vi "GetXL_SheetNames.vi"(8 "error in (no error)":errorcluster, 11 "Refnum Cluster In":T1) -> (0 "error out":errorcluster, 2 "SheetNames(\"\")":string[](array[string]), 3 "Refnum Cluster Out":T1)   [LabVIEW 2015]
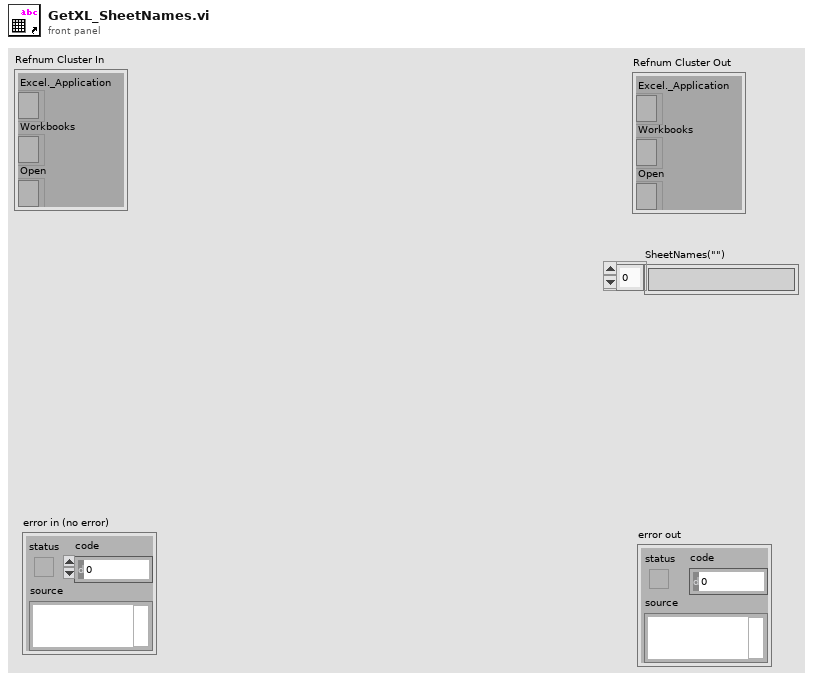
[diagram p1: front panel]
types:
  T1 = cluster{"Excel._Application":refnum<k7>, "Workbooks":refnum<k7>, "Open":refnum<k7>}
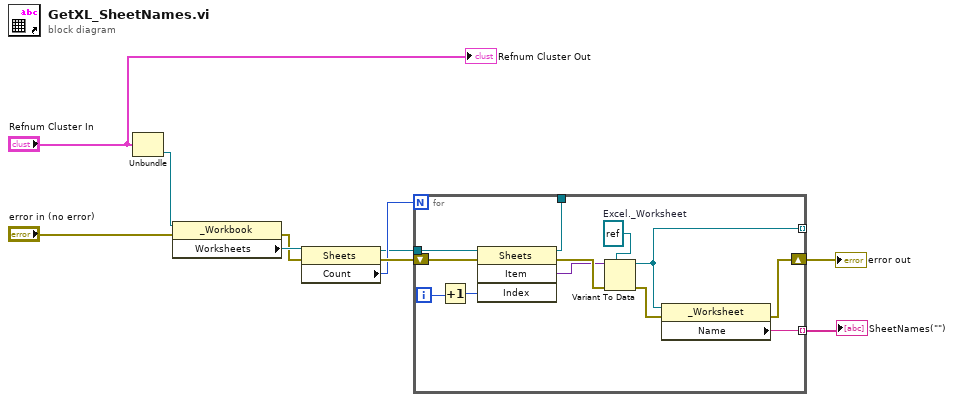
[diagram p0: block diagram]
diagram:
  n1 = Unbundle("Refnum Cluster In") -> ("Open"=w9:refnum<k7>)  [unwired: 2 out]
  n2 = property class="_Workbook"(reference=w9, error in="error in (no error)") -> (error out=w5:errorcluster, "Worksheets"=w6:refnum<k7>)  [unwired: 1 out]
  n3 = property class="Sheets"(reference=w6, error in=w5) -> (reference out=w2:refnum<k7>, error out=w4:errorcluster, "Count"=w3:i32)
  n4 = for {
    N: w3 -> [_]
    tunnel: [w22] -> _
    shift-right: [w16] -> w10
    shift-left: w4 -> [w18]
    tunnel: [w15] -> _ mode=indexing
    tunnel: [w14] -> w1 mode=indexing
    tunnel: w2 -> [w13]
    i -> [w12]
    w20 = refnum<k7> refnum  # Excel._Worksheet
    n5 = Increment(x=w12) -> (x+1=w11:i32)
    n6 = invoke class="Sheets" method="Item"(reference=w13, error in=w18, "Index"=w11) -> (reference out=w22:refnum<k7>, error out=w21:errorcluster, "Item"=w19:variant)  [unwired: 1 in, 1 out]
    n7 = Variant To Data(error in=w21, type=w20, Variant=w19) -> (data=w15:refnum<k7>, error out=w17:errorcluster)
    n8 = property class="_Worksheet"(reference=w15, error in=w17) -> (error out=w16:errorcluster, "Name"=w14:string)  [unwired: 1 out]
  }
  "error out" <- w10
  "SheetNames(\"\")" <- w1
  "Refnum Cluster Out" <- "Refnum Cluster In"
